vi "test code emballage_ZEBRA_RS232.vi"() -> ()   [LabVIEW 2011]
uses:
  <vilib>/Instr/_visa.llb/VISA Configure Serial Port (Instr).vi
panel:
  in  "Lecture ?":bool
  in  "Param RS232 2":T1={"VISA resource name"="COM4", "baud rate"=9600, "data bits"=8, "parity"=0, "stop bits"=10, "flow control"=1, "delay before read (ms)"=500} {"data bits" min=5 max=8 step=1; "parity" items=["Aucune", "Impaire", "Paire", "Marque", "Espace"]; "stop bits" items=["1.0"=10, "1.5"=15, "2.0"=20]; "flow control" items=["Aucune"=0, "XON/XOFF"=1, "RTS/CTS"=2, "DTR/DSR"=4]}
  in  "chaine a ecrire":string="^XA\n^KL3\n^SC9600,8,N,1,,N\n^PRA\n^LL1428\n^ML888\n^MMC\n^LH300,90\n\n\r\r^AFB,1,1^FT0,940^FDDestinataire : EMS Electro Medical System^FS\r^AFB,1,1^FT40,940^FDN§ commande : CF-08-0253/2^FS\r^AFB,1,1^FT80,940^FDQuantit‚ : 25/25^FS\r^AFB,1,1^FT120,940^FDVotre r‚f. : EL-360^FS\r^AFB,1,1^FT200,940^FDN§ valves :^FS\r^AFB,1,1^FT235,905^FD(P/N)^FS\r\r^FT630,30\n^BY2,2.0\n^BCI,80,N,N,N\n^FD MK01852  09 08010802 50^FS\r^A0I,30,30^FT485,0^FD MK01852  09 08010802 50^FS\r\r^A0B,24,24^FT200,750^FD 08010001,  08010002,  08010003,  08010004,  08010004^FS\r^A0B,24,24^FT225,750^FD 08010005,  08010006,  08010007,  08010008,  08010004^FS\r^A0B,24,24^FT250,750^FD 08010009,  08010010,  08010011,  08010012,  08010004^FS\r^A0B,24,24^FT275,750^FD 08010013,  08010014,  08010015,  08010016,  08010004^FS\r^A0B,24,24^FT300,750^FD 08010017,  08010018,  08010019,  08010020,  08010004^FS\r^A0B,24,24^FT325,750^FD 08010022,  08010030,  08010099,  08020006,  08010004^FS\r^A0B,24,24^FT350,750^FD 08010022,  08010030,  08010099,  08020006,  08010004^FS\r^A0B,24,24^FT375,750^FD 08010022,  08010030,  08010099,  08020006,  08010004^FS\r^A0B,24,24^FT400,750^FD 08010022,  08010030,  08010099,  08020006,  08010004^FS\r^A0B,24,24^FT425,750^FD 08010022,  08010030,  08010099,  08020006,  08010004^FS\r\r^FT465,940\n^GB0,800,3^FS\n\n^FT650,940\n^BXB,6,0\n^FD12-216C-04521 EQIFIL 417mA 14.4ohm;03838/08-01.07.01;1/1^FS\r^AFB,1,1^FT525,760^FDN§ article FAS :^FS\r^A0B,30,30^FT560,760^FD12-216C-04521 EQIFIL 417mA 14.4ohm^FS\r^AFB,1,1^FT595,760^FDN§ commande FAS :^FS\r^A0B,30,30^FT630,760^FD03838/08-01.07.01^FS\r^AFB,1,1^FT665,760^FDCarton : ^FS\r^A0B,30,30^FT665,616^FD1/1^FS\r\r^PQ1\n^XZ\r"
  out "chaine lue":string="\n"
  in  "Param RS232":T1={"VISA resource name"="COM4", "baud rate"=9600, "data bits"=8, "parity"=0, "stop bits"=10, "flow control"=0, "delay before read (ms)"=500} {"data bits" min=5 max=8 step=1; "parity" items=["Aucune", "Impaire", "Paire", "Marque", "Espace"]; "stop bits" items=["1.0"=10, "1.5"=15, "2.0"=20]; "flow control" items=["Aucune"=0, "XON/XOFF"=1, "RTS/CTS"=2, "DTR/DSR"=4]}
  # "Grande etiquette - 1 code bar 2D + scan"
  # "Grande etiquette - 1 code bar 2D"
  # "ZB\nUS\nq592\nD7\nN\nR166,48\nI8,12,001\nA504,828,2,1,1,1,N,\"FASmedic s.a.\"\nA504,812,2,1,1,1,N,\"Zone industrielle\"\nA504,796,2,1,1,1,N,\"CH-1607 Pal‚zieux-Gare\"\nA504,780,2,1,1,1,N,\"T‚l.+41(0)21 907 79 71\"\nA504,764,2,1,1,1,N,\"www.fasmedic.com\"\nA34,712,3,2,1,1,N,\"Destinataire:EMS Electro Medical System\"\nA74,712,3,2,1,1,N,\"Nшcommande:CF-08-0253/2\"\nA114,712,3,2,1,1,N,\"Carton:1/2\"\nA154,712,3,2,1,1,N,\"Quantit‚:50/100\"\nA194,712,3,2,1,1,N,\"Votre ref.:EL-360\"\nLO258,112,2,600\nb404,112,D,4,\"12-216C-04521 EQIFIL 417mA 14.4ohm     03838/08-07.01.01\"\nA318,712,3,2,1,1,N,\"Nшarticle FAS:\"\nA358,712,3,3,1,1,N,\"12-216C-04521 EQIFIL 417mA 14.4ohm\"\nA398,712,3,2,1,1,N,\"Nшcommande FAS:\"\nA438,712,3,3,1,1,N,\"03838/08-07.01.01\"\nB318,64,2,3,1,2,56,N,\"EL-360 03 08010801\"\nA318,0,2,3,1,1,N,\"EL-360 03 08010801\"\nGW265,824,32,61,яяяяяяяяяяяяяяяяяяяяяяяяяяяяяяяЏяяяяяяяяяяяяяяяяяяяяяяяяяяяяяяюяяяяяяяяяяяяяяяяяяяяяяяяяяяяяяшяяяяяяяяяяяяяяяяяяяяяяяяяяяяяяАяяяяяяяяяяяяяяяяяяяяяяяяяяяяяяяяяяяяяяяяяяяяяяяяяяяяяяяяяяяяяяяяяяяяяяяяяяяяяяяяяяяяяяяяяюяяяяяяяяяяяяяяяяяяяяяяяяяяяяяюяяяяяяяяяяяяяяяяяяяяяяяяяяяяяюяяяяяяяяяяяяяяяяяяяяяяяяяяяяяьяяяяяяяяяяяяяяяяяяяяяяяяяяяяяьяяяяяяяяяяяяяяяяяяяяяяяяяяяяяшяЃяяяяьяяяяяяаяяяЂ?яяяяяяяшюП<ярьящяуя?Аяю8ш>П0x?БрьящяуьАяь0щяЏП#яЏь|ящяушАяшpуяЗП'яЏю<ящяурАяр`гягПяЏ?яящяуарАшяаазяуПяЗ?яњящяуашАьяЂАЗяуПяж?яњящяуашАьяАПяыПяжяЬящяуаяяАья~АяящПязяяМящяуаяяАшяЂяящП?язяяМящяуаяАаяЂяящП?ячяяМящяур?АяЂ?яящП?яцящяурАяА?яящП?яцящяушАяаяящП?яжяМящяуяАяряящПяжяЬящяуярАяяряяыПяжяњящягяяаАяяяшяПяуПяж?яњящягррАяяяяяяяяяяЗяуПяЗ?яясягррАшяяяяяяязягПяП?я>ясягрраряЂягязП'яЏџю>аяГраяЂ0ясяЏП#я‡ь~?А“шря0яшяП1ь?ГряЊ3ьшюpяь?П8аяЂsьью`яяЃяя?ѓяюяаяГяяАяяАяяьаяяяяя?яяяяяяяяяяяяяяяяяяьАяяяяя?яяяяяяяяяяяяяяяяяюьАяяяяя?яяяяяяяяяяяяяяяяяюшАяяяяя?яяяяяяяяяяяяяяяяяьшЂяяяяП?яяяяяяяяяяяяяяяяярЂяяяяП?яяяяяяяяяяяяяяяяяяр?яяяяП?яяяяяяяяяяяяяяяяяяр?яяяяП?яяяяяяяяяяяяяяяяяяаяяяяП?яяяяяяяяяяяяяяяяяяаяяяяяяяяяяяяяяяяяяяяяяяяАяяяяяяяяяяяяяяяяяяяяяяяяяяяАяяяяяяяяяяяяяяяяяяяяяяяяяяяЂяяяяяяяяяяяяяяяяяяяяяяяяяяяяяЂяяяяяяяяяяяяяяяяяяяяяяяяяяяяяЂ?яяяяяяяяяяяяяяяяяяяяяяяяяяяяяЂ?яяяяяяяяяяяяяяяяяяяяяяяяяяяяяЂ?яяяяяяяяяяяяяяяяяяяяяяяяяяяяяЂяяяяяяяяяяяяяяяяяяяяяяяяяяяяяАяяяяяяяяяяяяяяяяяяяяяяяяяяяяяаяяяяяяяяяяяяяяяяяяяяяяяяяяяяяяаяяяяяяяяяяяяяяяяяяяяяяяяяяяяяяряяяяяяяяяяяяяяяяяяяяяяяяяяяяяяр?яяяяяяяяяяяяяяяяяяяяяяяяяяяяяяшяяяяяяяяяяяяяяяяяяяяяяяяяяяяяящяяяяяя\nP1"
  # "PROTO GmbH normal"
  # "^XA\n^KL3\n^SC9600,8,N,1,,N\n^PRA\n^LL1428\n^ML888\n^MMC\n^LH300,90\n\n\n\n^AFB,1,1^FT0,940^FDDestinataire : EMS Electro Medical System^FS\n^AFB,1,1^FT40,940^FDN§ commande : CF-08-0253/2^FS\n^AFB,1,1^FT80,940^FDQuantit‚ : 25/25^FS\n^AFB,1,1^FT120,940^FDVotre r‚f. : EL-360^FS\n^AFB,1,1^FT200,940^FDN§ valves :^FS\n^AFB,1,1^FT235,905^FD(P/N)^FS\n\n^FT630,30\n^BY2,2.0\n^BCI,80,N,N,N\n^FD MK01852  09 08010802 50^FS\n^A0I,30,30^FT485,0^FD MK01852  09 08010802 50^FS\n\n^A0B,24,24^FT200,750^FD 08010001,  08010002,  08010003,  08010004,  08010004^FS\n^A0B,24,24^FT225,750^FD 08010005,  08010006,  08010007,  08010008,  08010004^FS\n^A0B,24,24^FT250,750^FD 08010009,  08010010,  08010011,  08010012,  08010004^FS\n^A0B,24,24^FT275,750^FD 08010013,  08010014,  08010015,  08010016,  08010004^FS\n^A0B,24,24^FT300,750^FD 08010017,  08010018,  08010019,  08010020,  08010004^FS\n^A0B,24,24^FT325,750^FD 08010022,  08010030,  08010099,  08020006,  08010004^FS\n^A0B,24,24^FT350,750^FD 08010022,  08010030,  08010099,  08020006,  08010004^FS\n^A0B,24,24^FT375,750^FD 08010022,  08010030,  08010099,  08020006,  08010004^FS\n^A0B,24,24^FT400,750^FD 08010022,  08010030,  08010099,  08020006,  08010004^FS\n^A0B,24,24^FT425,750^FD 08010022,  08010030,  08010099,  08020006,  08010004^FS\n\n^FT465,940\n^GB0,800,3^FS\n\n^FT650,940\n^BXB,6,0\n^FD12-216C-04521 EQIFIL 417mA 14.4ohm;03838/08-01.07.01;1/1^FS\n^AFB,1,1^FT525,760^FDN§ article FAS :^FS\n^A0B,30,30^FT560,760^FD12-216C-04521 EQIFIL 417mA 14.4ohm^FS\n^AFB,1,1^FT595,760^FDN§ commande FAS :^FS\n^A0B,30,30^FT630,760^FD03838/08-01.07.01^FS\n^AFB,1,1^FT665,760^FDCarton : ^FS\n^A0B,30,30^FT665,616^FD1/1^FS\n\n^PQ1\n^XZ"
  # "PROTO GmbH RETOUR"
  # "Test des polices"
  # "^XA\n^KL3\n^SC9600,8,N,1,,N\n^PRA\n^LL1428\n^ML888\n^MMC\n^LH300,90\n\n\n\n^AFB,1,1^FT0,940^FDDestinataire : EMS Electro Medical System^FS\n^AFB,1,1^FT40,940^FDN§ commande : CF-08-0253/2^FS\n^AFB,1,1^FT80,940^FDQuantit‚ : 25/25^FS\n^AFB,1,1^FT120,940^FDVotre r‚f. : EL-360^FS\n^AFB,1,1^FT200,940^FDN§ valves :^FS\n^AFB,1,1^FT235,905^FD(P/N)^FS\n\n^AVI,1,1^FT370,26^FDRETOUR^FS\n\n^A0B,24,24^FT200,750^FD 08010001,  08010002,  08010003,  08010004^FS\n^A0B,24,24^FT225,750^FD 08010005,  08010006,  08010007,  08010008^FS\n^A0B,24,24^FT250,750^FD 08010009,  08010010,  08010011,  08010012^FS\n^A0B,24,24^FT275,750^FD 08010013,  08010014,  08010015,  08010016^FS\n^A0B,24,24^FT300,750^FD 08010017,  08010018,  08010019,  08010020^FS\n^A0B,24,24^FT325,750^FD 08010022,  08010030,  08010099,  08020006^FS\n^A0B,24,24^FT350,750^FD 08010022^FS\n^A0B,24,24^FT375,750^FD^FS\n^A0B,24,24^FT400,750^FD^FS\n^A0B,24,24^FT425,750^FD^FS\n\n^FT465,940\n^GB0,800,3^FS\n\n^FT650,940\n^BXB,6,0\n^FD12-216C-04521 EQIFIL 417mA 14.4ohm;R03838/08-01.07.01;1/1^FS\n^AFB,1,1^FT525,760^FDN§ article FAS :^FS\n^A0B,30,30^FT560,760^FD12-216C-04521 EQIFIL 417mA 14.4ohm^FS\n^AFB,1,1^FT595,760^FDN§ commande FAS :^FS\n^A0B,30,30^FT630,760^FDR03838/08-01.07.01^FS\n^AFB,1,1^FT665,760^FDCarton : ^FS\n^A0B,30,30^FT665,616^FD1/1^FS\n\n^PQ1\n^XZ"
  # "^XA\n^KL3\n^SC9600,8,N,1,,N\n^PRA\n^LL976\n^ML592\n^LH50,25\n\n^AFB,1,1^FT20,704^FDDestinataire :  EMS Electro Medical System^FS\n^ADB,1,1^FT50,704^FDDestinataire :  EMS Electro Medical System^FS\n^AQB,1,1^FT80,704^FDDestinataire :  EMS Electro Medical System^FS\n^APB,1,1^FT110,704^FDDestinataire :  EMS Electro Medical System^FS\n^ARB,1,1^FT140,704^FDDestinataire :  EMS Electro Medical System^FS\n^A0B,16,16^FT170,704^FDDestinataire :  EMS Electro Medical System^FS\n^A0B,18,18^FT200,704^FDDestinataire :  EMS Electro Medical System^FS\n^A0B,20,20^FT230,704^FDDestinataire :  EMS Electro Medical System^FS\n^A0B,22,22^FT260,704^FDDestinataire :  EMS Electro Medical System^FS\n^A0B,24,24^FT290,704^FDDestinataire :  EMS Electro Medical System^FS\n^A0B,26,26^FT320,704^FDDestinataire :  EMS Electro Medical System^FS\n^A0B,28,28^FT350,704^FDDestinataire :  EMS Electro Medical System^FS\n^A0B,30,30^FT380,704^FDDestinataire :  EMS Electro Medical System^FS\n\n^PQ1\n^XZ"
  # "^XA\n^KL3\n^SC9600,8,N,1,,N\n^PRA\n^LL1428\n^ML888\n^MMC\n^LH300,90\n\n\n\n^AFB,1,1^FT0,940^FDDestinataire : EMS Electro Medical System^FS\n^AFB,1,1^FT40,940^FDN§ commande : CF-08-0253/2^FS\n^AFB,1,1^FT80,940^FDQuantit‚ : 25/25^FS\n^AFB,1,1^FT120,940^FDVotre r‚f. : EL-360^FS\n^AFB,1,1^FT200,940^FDN§ valves :^FS\n^AFB,1,1^FT235,905^FD(P/N)^FS\n\n^AVI,1,1^FT370,26^FDRETOUR^FS\n\n^A0B,24,24^FT200,750^FD 08010001,  08010002,  08010003,  08010004^FS\n^A0B,24,24^FT225,750^FD 08010005,  08010006,  08010007,  08010008^FS\n^A0B,24,24^FT250,750^FD 08010009,  08010010,  08010011,  08010012^FS\n^A0B,24,24^FT275,750^FD 08010013,  08010014,  08010015,  08010016^FS\n^A0B,24,24^FT300,750^FD 08010017,  08010018,  08010019,  08010020^FS\n^A0B,24,24^FT325,750^FD 08010022,  08010030,  08010099,  08020006^FS\n^A0B,24,24^FT350,750^FD 08010022^FS\n^A0B,24,24^FT375,750^FD^FS\n^A0B,24,24^FT400,750^FD^FS\n^A0B,24,24^FT425,750^FD^FS\n\n^FT465,940\n^GB0,800,3^FS\n\n^FT650,940\n^BXB,6,0\n^FD12-216C-04521 EQIFIL 417mA 14.4ohm;R03838/08-01.07.01;1/1^FS\n^AFB,1,1^FT525,760^FDN§ article FAS :^FS\n^A0B,30,30^FT560,760^FD12-216C-04521 EQIFIL 417mA 14.4ohm^FS\n^AFB,1,1^FT595,760^FDN§ commande FAS :^FS\n^A0B,30,30^FT630,760^FDR03838/08-01.07.01^FS\n^AFB,1,1^FT665,760^FDCarton : ^FS\n^A0B,30,30^FT665,616^FD1/1^FS\n\n^PQ1\n^XZ"
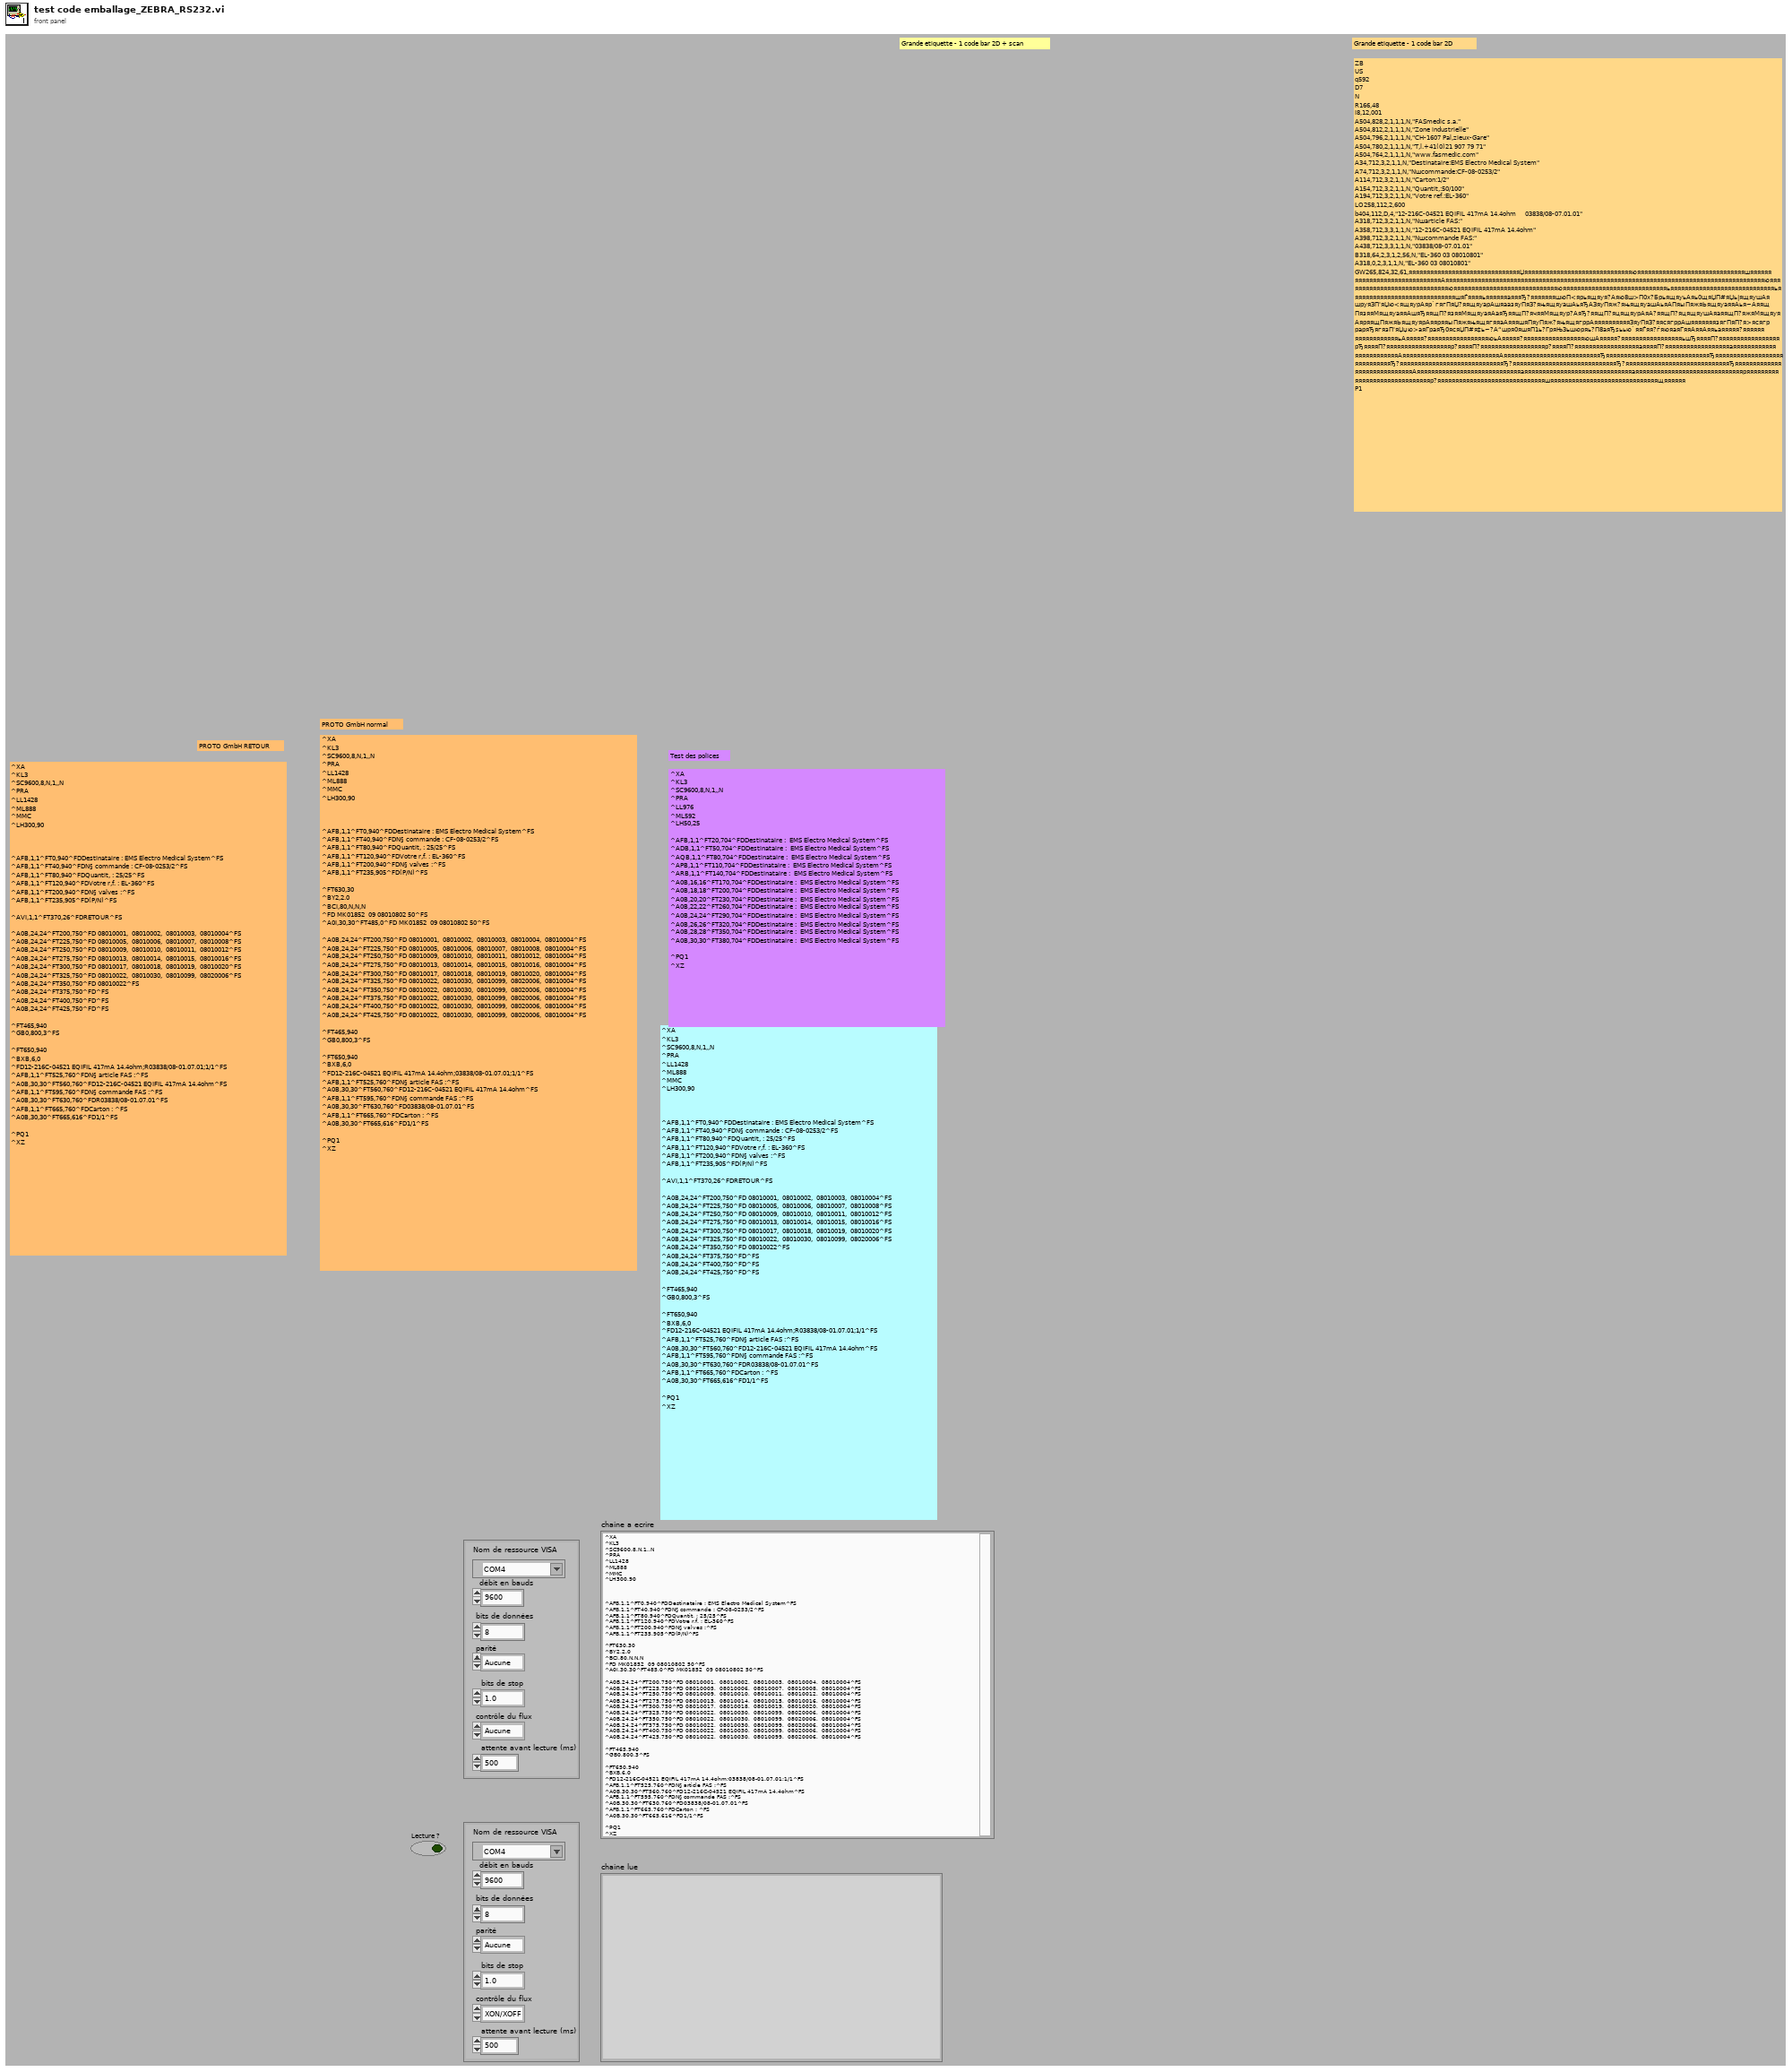
[diagram p1: front panel]
types:
  T1 = cluster{"VISA resource name":refnum<visa-resource-name>, "baud rate":u32, "data bits":u16, "parity":u16, "stop bits":u16, "flow control":u16, "delay before read (ms)":u32}
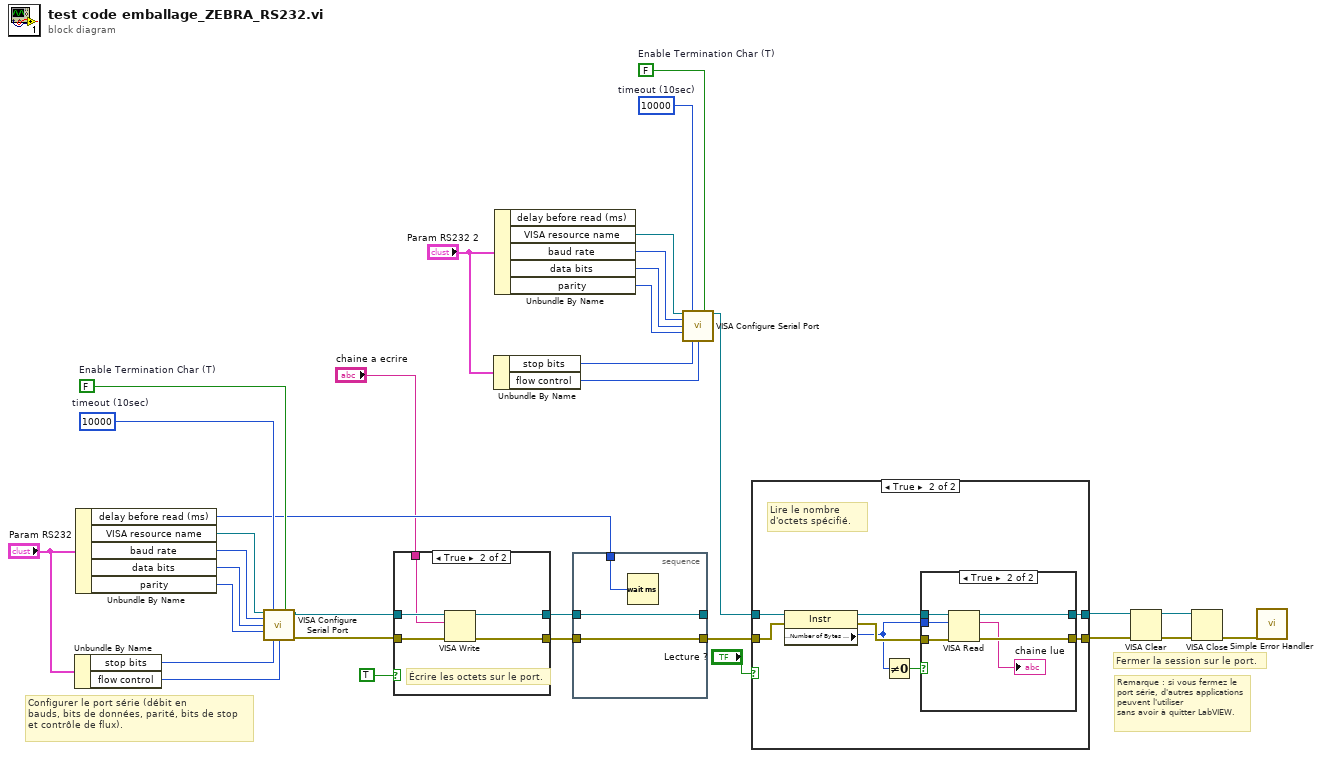
[diagram p0: block diagram]
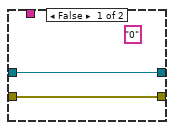
[diagram p2: hidden frame]
diagram:
  w6 = FALSE  # Enable Termination Char (T)
  w7 = u32 10000  # timeout (10sec)
  w32 = FALSE  # Enable Termination Char (T)
  w33 = u32 10000  # timeout (10sec)
  # "Remarque : si vous fermez le port série, d'autres applications peuvent l'utiliser\nsans avoir à quitter LabVIEW."
  # "Fermer la session sur le port."
  # "Configurer le port série (débit en\nbauds, bits de données, parité, bits de stop\net contrôle de flux)."
  n1 = Unbundle By Name("Param RS232") -> ("stop bits"=w26:u16, "flow control"=w25:u16)
  n2 = Unbundle By Name("Param RS232") -> ("delay before read (ms)"=w18:u32, "VISA resource name"=w31:refnum<visa-resource-name>, "baud rate"=w30:u32, "data bits"=w29:u16, "parity"=w28:u16)
  n3 = call-poly "VISA Configure Serial Port"("VISA resource name"=w31, "timeout (10sec)"=w33, "Enable Termination\nChar (T)"=w32, "baud rate (9600)"=w30, "data bits (8)"=w29, "parity (0:none)"=w28, "stop bits (10: 1 bit)"=w26, "flow control (0:none)"=w25) -> ("VISA resource name out"=w17:refnum<visa-resource-name>, "error out"=w16:errorcluster)  [unwired: 6 in]
  n4 = case shown="True" TRUE {
    tunnel: [w35 w40] -> w23
    tunnel: w17 -> [w34 w39]
    tunnel: w16 -> [w35 w38]
    tunnel: [w34 w37] -> w21
    tunnel: "chaine a ecrire" -> [_ w36]
    frame False {
      (unwired) "0" ("string to write")
    }
    frame True {
      # "Écrire les octets sur le port."
      n5 = VISA Write(VISA resource name=w39, write buffer=w36, error in (no error)=w38) -> (VISA resource name out=w37:refnum<visa-resource-name>, error out=w40:errorcluster)  [unwired: 1 out]
    }
  }
  n6 = Unbundle By Name("Param RS232 2") -> ("stop bits"=w9:u16, "flow control"=w8:u16)
  n7 = Unbundle By Name("Param RS232 2") -> ("VISA resource name"=w14:refnum<visa-resource-name>, "baud rate"=w13:u32, "data bits"=w12:u16, "parity"=w11:u16)  [unwired: 1 out]
  n8 = stacked-sequence {
    tunnel: w23 -> [w43]
    tunnel: [w43] -> w22
    tunnel: w21 -> [w42]
    tunnel: [w42] -> _
    tunnel: w18 -> [w41]
    frame #0 {
      n9 = Wait (ms)(milliseconds to wait=w41) -> ()  [unwired: 1 out]
    }
  }
  n10 = call-poly "VISA Configure Serial Port"("VISA resource name"=w14, "timeout (10sec)"=w7, "Enable Termination\nChar (T)"=w6, "baud rate (9600)"=w13, "data bits (8)"=w12, "parity (0:none)"=w11, "stop bits (10: 1 bit)"=w9, "flow control (0:none)"=w8) -> ("VISA resource name out"=w5:refnum<visa-resource-name>)  [unwired: 6 in, 1 out]
  n11 = case shown="True" "Lecture ?" {
    tunnel: w22 -> [w45 w49]
    tunnel: [w45 w53] -> w3
    tunnel: [w44 w52] -> w4
    tunnel: w5 -> [w44 w51]
    frame False {
    }
    frame True {
      # "Lire le nombre d'octets spécifié."
      n12 = property class="Instr"(reference=w51, error in=w49) -> (reference out=w50:refnum<visa-resource-name>, error out=w48:errorcluster, "Serial Settings:Number of Bytes at Serial Port"=w46:u32)
      n13 = Not Equal To 0?(x=w46) -> (x != 0?=w47:bool)
      n14 = case shown="True" w47 {
        tunnel: [w55 w61] -> w53
        tunnel: [w54 w60] -> w52
        tunnel: w50 -> [w54 w59]
        tunnel: w48 -> [w55 w58]
        tunnel: w46 -> [_ w56]
        frame False {
        }
        frame True {
          n15 = VISA Read(VISA resource name=w59, byte count=w56, error in (no error)=w58) -> (VISA resource name out=w60:refnum<visa-resource-name>, read buffer=→"chaine lue":string, error out=w61:errorcluster)  [unwired: 1 out]
        }
      }
    }
  }
  n16 = VISA Clear(VISA resource name=w4, error in (no error)=w3) -> (VISA resource name out=w1:refnum<visa-resource-name>, error out=w2:errorcluster)
  n17 = VISA Close(VISA resource name=w1, error in (no error)=w2) -> (error out=w24:errorcluster)
  n18 = call <vilib>:"Simple Error Handler.vi"("error in (no error)"=w24) -> ()  [unwired: 4 in, 5 out]
